vi "Right Joystick Button Map.vi"(1 "Joystick Name":string="Right Joystick") -> (0 "Actions":T1={"Precision Mode?"=TRUE, "Left-Right"=0.0, "Shift Desired"=TRUE, "Manual Shooter Speed"=0.0})   [LabVIEW 2012]
uses:
  <vilib>/Rock Robotics/WPI/Joystick/WPI_JoystickGetSetRefNum.vi
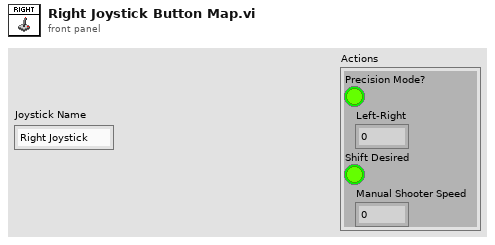
[diagram p1: front panel]
types:
  T1 = cluster{"Precision Mode?":bool, "Left-Right":dbl, "Shift Desired":bool, "Manual Shooter Speed":dbl}
  T2 = typedef "WPI_JoystickDevRef.ctl" = cluster{"Device":T3}
  T3 = typedef "WPI_JoystickDeviceEnum.ctl" = enum16{"USB 1", "USB 2", "USB 3", "USB 4", "Kinect 1", "Kinect 2"}
  T4 = typedef "WPI_JoystickButtonState.ctl" = cluster{"Button 1":bool, "Button 2":bool, "Button 3":bool, "Button 4":bool, "Button 5":bool, "Button 6":bool, "Button 7":bool, "Button 8":bool, "Button 9":bool, "Button 10":bool, "Button 11":bool, "Button 12":bool}
  T5 = cluster{"axis 1 (x)":dbl, "axis 2 (y)":dbl, "axis 3 (throttle)":dbl, "axis 4":dbl, "axis 5":dbl, "axis 6":dbl}
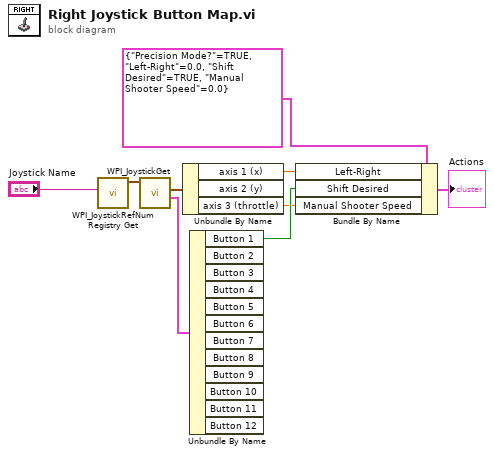
[diagram p0: block diagram]
diagram:
  n1 = call <vilib>:"WPI_JoystickRefNum Registry Get.vi"("refnum name"="Joystick Name") -> ("JoystickDevRef"=w9:T2)  [unwired: 1 in, 9 out]
  n2 = call <vilib>:"WPI_JoystickGet.vi"("JoystickDevRef"=w9) -> ("Buttons"=w6:T4, "Axes"=w7:T5)  [unwired: 1 in, 4 out]
  n3 = Unbundle By Name(w7) -> ("axis 1 (x)"=w4:dbl, "axis 3 (throttle)"=w1:dbl)  [unwired: 1 out]
  n4 = Unbundle By Name(w6) -> ("Button 1"=w3:bool)  [unwired: 11 out]
  n5 = Bundle By Name(cluster=T1 {"Precision Mode?"=TRUE, "Left-Right"=0.0, "Shift Desired"=TRUE, "Manual Shooter Speed"=0.0}, "Left-Right"=w4, "Shift Desired"=w3, "Manual Shooter Speed"=w1) -> (→"Actions":T1)
